vi "Task02.vi"() -> ()   [LabVIEW 2017]
panel:
  out "Number Array":dbl[](array[numeric])
  in  "stop":bool
  in  "Switch Array":bool[](array[boolean])
  out "LED Array":bool[](array[boolean])
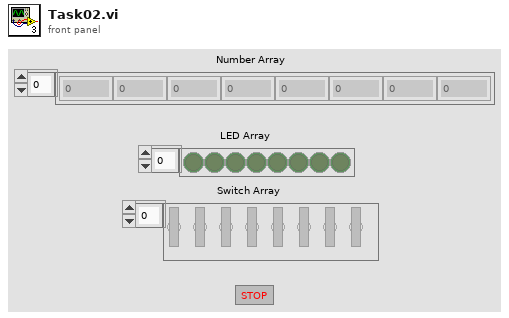
[diagram p1: front panel]
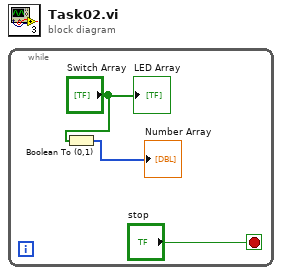
[diagram p0: block diagram]
diagram:
  n1 = while {
    stop <- "stop" stop-if-true
    n2 = Boolean To (0,1)(Boolean="Switch Array") -> (0, 1=→"Number Array":i16[])
    "LED Array" <- "Switch Array"
  }
